vi "G#Object_ExternalCreateProcess.vi"(0 "occurrence":refnum<k4>, 5 "error in (no error)":errorcluster) -> (19 "error out":errorcluster)   [LabVIEW 2020, in "G#Object.lvclass"]
doc: "This is an external create process that will create an own all objects. It is stopped when running the garbage collector."
uses:
  <vilib>/addons/_AddQ/G#Object/G#Object.lvclass
  <vilib>/addons/_AddQ/G#Object/utils/G#Object_Event.ctl
  <vilib>/addons/_AddQ/G#Object/utils/G#Object_EventType.ctl
  <vilib>/addons/_AddQ/G#Object/utils/G#Object_ObjectInfoType.ctl
  <vilib>/addons/_AddQ/G#Object/utils/G#Object_CreateMethod.ctl
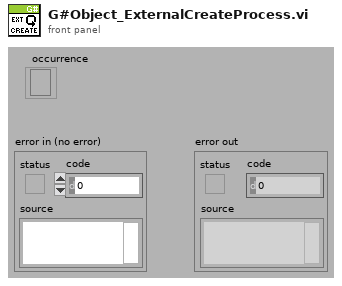
[diagram p1: front panel]
types:
  T1 = typedef "G#Object.lvclass/G#Object_Event.ctl" = cluster{"EventType":T2, "ObjectInfo":T3, "Ref":refnum<class "G#Object.lvclass">, "Time Stamp":timestamp, "LogText":string, "Parameters":variant[]}
  T2 = typedef "G#Object.lvclass/G#Object_EventType.ctl" = enum16{"Created new", "Looked up existing", "Deleted", "Forced delete", "Not deleted", "Garbage collected", "Cleared", "User", "Error", "External create object", "External create class attributes", "Created class attributes", "Run constructor", "Run constructor done", "Run open method", "Run open method done"}
  T3 = typedef "G#Object.lvclass/G#Object_ObjectInfoType.ctl" = cluster{"ObjectName":string, "ObjectID":u32, "Users":i32, "Counter":bool, "AttributeRefs":u32[], "FullClassName":string, "ClassName":string, "CreateMethod":T4, "GenericDestructorExists":bool, "Owner":string}
  T4 = typedef "G#Object.lvclass/G#Object_CreateMethod.ctl" = enum16{"Create", "Create or look up existing", "Look up existing"}
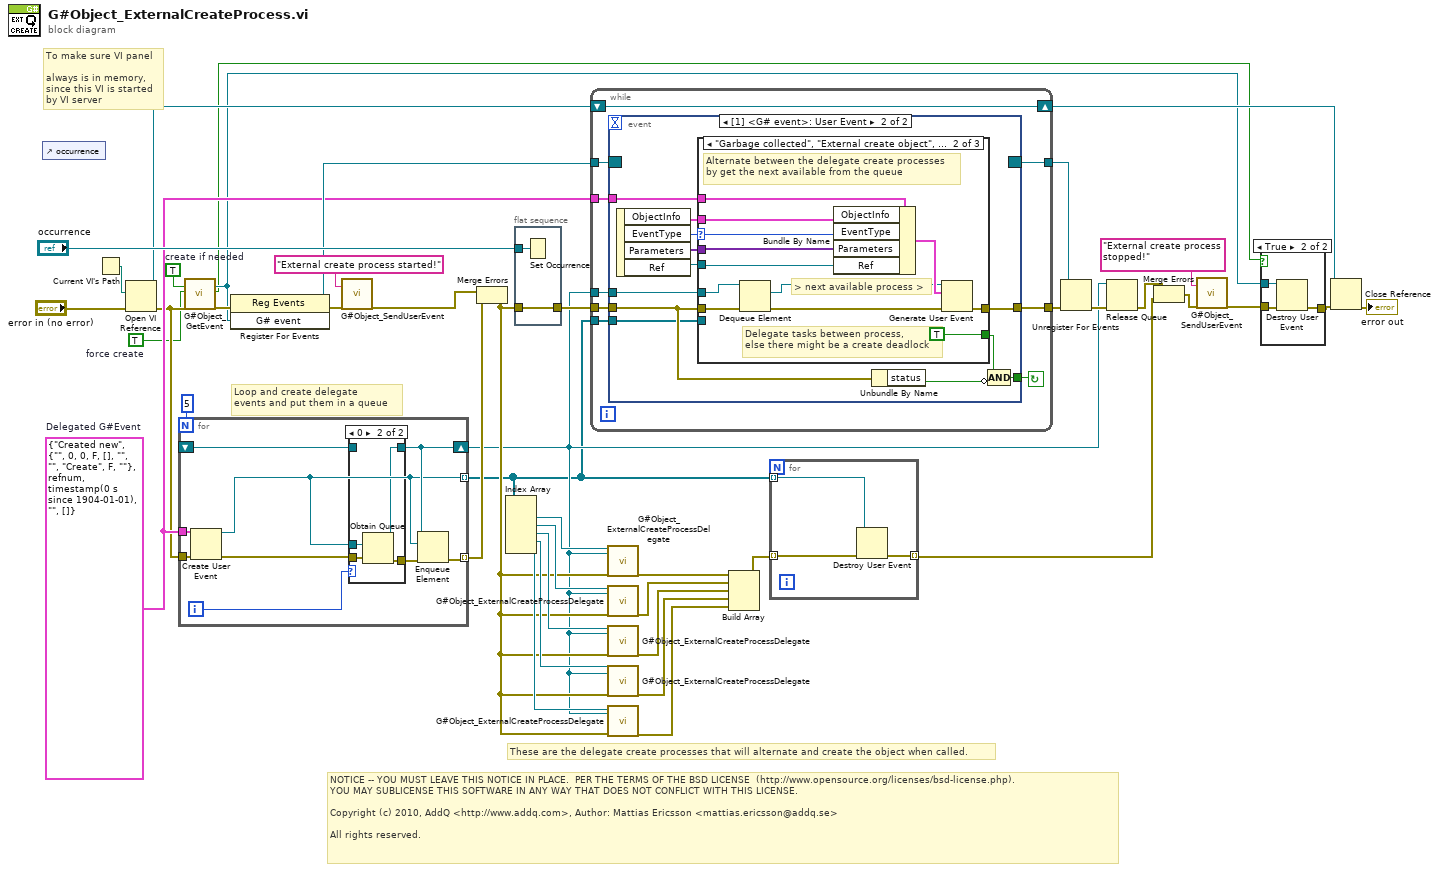
[diagram p0: block diagram]
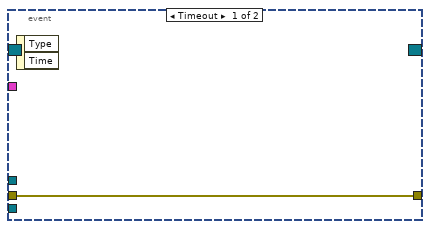
[diagram p4: hidden frame]
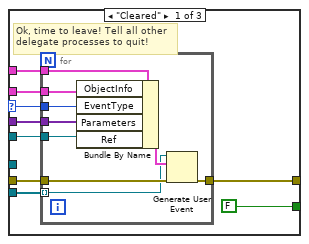
[diagram p5: hidden frame]
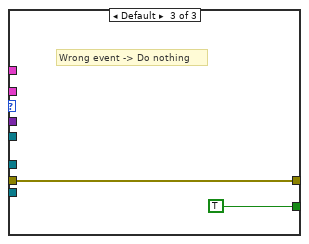
[diagram p6: hidden frame]
diagram:
  w2 = TRUE  # force create
  w30 = T1 {"EventType"=enum."Created new", "ObjectInfo"={"ObjectName"="", "ObjectID"=0, "Users"=0, "Counter"=FALSE, "AttributeRefs"=[], "FullClassName"="", "ClassName"="", "CreateMethod"=enum."Create", "GenericDestructorExists"=FALSE, "Owner"=""}, "Ref"=refnum, "Time Stamp"=timestamp(0 s since 1904-01-01), "LogText"="", "Parameters"=[]}  # Delegated G#Event
  w40 = TRUE  # create if needed
  # "Loop and create delegate\nevents and put them in a queue"
  # "These are the delegate create processes that will alternate and create the object when called."
  # "To make sure VI panel\n\nalways is in memory,\nsince this VI is started\nby VI server"
  # "NOTICE -- YOU MUST LEAVE THIS NOTICE IN PLACE.  PER THE TERMS OF THE BSD LICENSE  (http://www.opensource.org/licenses/bsd-license.php).\nYOU MAY SUBLICENSE THIS SOFTWARE IN ANY WAY THAT DOES NOT CONFLICT WITH THIS LICENSE.\n\nCopyright (c) 2010, AddQ <http://www.addq.com>, Author: Mattias Ericsson <mattias.ericsson@addq.se>\n\nAll rights reserved."
  n1 = control-ref of="occurrence"() -> ()  [unwired: 1 out]
  n2 = Current VI's Path() -> (path=w35:path)
  n3 = Open VI Reference(vi path=w35, error in (no error)="error in (no error)") -> (vi reference=w36:refnum<vi>, error out=w29:errorcluster)  [unwired: 4 in]
  n4 = for {
    N: 5 -> [_]
    tunnel: w30 -> [w52]
    tunnel: w29 -> [w51]
    tunnel: [w46] -> w1 mode=indexing
    tunnel: [w45] -> w24 mode=indexing
    shift-right: [w47] -> w8
    shift-left: _ -> [w49]
    i -> [w50]
    n5 = Create User Event(user event datatype=w52, error in=w51) -> (user event=w46:refnum<user-event>, error out=w44:errorcluster)
    n6 = case shown="0" w50 {
      tunnel: w44 -> [w53 w58]
      tunnel: w46 -> [_ w57]
      tunnel: [w54 w56] -> w47
      tunnel: w49 -> [w54 _]
      tunnel: [w53 w55] -> w48
      frame Default {
      }
      frame 0 {
        n7 = Obtain Queue(element data type=w57, error in (no error)=w58) -> (queue out=w56:refnum<queue>, error out=w55:errorcluster)  [unwired: 3 in, 1 out]
      }
    }
    n8 = Enqueue Element(queue=w47, element=w46, error in (no error)=w48) -> (error out=w45:errorcluster)  [unwired: 1 in, 2 out]
  }
  n9 = call <vilib>:"G#Object_GetEvent.vi"("create if needed (T)"=w40, "force create (F)"=w2, "error in (no error)"=w29) -> ("G# event"=w4:refnum<user-event>, "created new"=w3:bool, "error out"=w39:errorcluster)  [unwired: 12 in, 2 out]
  n10 = register-events(error in=w39, w4) -> (reference out=w37:refnum<event-registration>, error out=w33:errorcluster)  [unwired: 1 in]
  n11 = call <vilib>:"G#Object_SendUserEvent.vi"("text"="External create process started!" ("Text"), "error in (no error)"=w33) -> ("error out"=w28:errorcluster)  [unwired: 16 in, 1 out]
  n12 = Merge Errors(w28, w24) -> (w13:errorcluster)
  n13 = Index Array(array=w1) -> (element #1=w18:refnum<user-event>, element #2=w17:refnum<user-event>, element #3=w16:refnum<user-event>, element #4=w15:refnum<user-event>, element #5=w14:refnum<user-event>)  [unwired: 5 in]
  n14 = flat-sequence {
    tunnel: "occurrence" -> [w60]
    tunnel: w13 -> [w59]
    tunnel: [w59] -> w12
    frame #0 {
      n15 = Set Occurrence(w60) -> ()
    }
  }
  n16 = while {
    tunnel: w12 -> [w69]
    tunnel: [w68] -> w31
    tunnel: w37 -> [w67]
    tunnel: [w66] -> w38
    shift-right: [w65] -> w34
    shift-left: w36 -> [w65]
    tunnel: w30 -> [w63]
    tunnel: w8 -> [w62]
    tunnel: w1 -> [w61]
    stop <- w64 continue-if-true
    n17 = event shown="[1] <G# event>: User Event" {
      selector: w67 -> [_ _]
      dyn-events: [_ _] -> w66
      timeout: _ -> [_ _]
      tunnel: w69 -> [w70 w80]
      tunnel: [w70 w82] -> w68
      tunnel: [_ w77] -> w64
      tunnel: w63 -> [_ w74]
      tunnel: w62 -> [_ w73]
      tunnel: w61 -> [_ w72]
      event Timeout {
        n18 = event-data() -> ()  [unwired: 1 in, 2 out]
      }
      event User Event {
        n19 = event-data() -> ("ObjectInfo"=w75:T3, "EventType"=w81:T2, "Parameters"=w76:variant[], "Ref"=w71:refnum<class "G#Object.lvclass">)  [unwired: 1 in]
        n20 = case shown="\"Garbage collected\", \"External create object\", \"External create class attributes\", \"Run constructor\", \"Run open method\"" w81 {
          selector: w81 -> [w88 w108 _]
          tunnel: w80 -> [w87 w105 w113]
          tunnel: [w90 w111 w113] -> w82
          tunnel: [FALSE TRUE TRUE] -> w78
          tunnel: w76 -> [w84 w107 _]
          tunnel: w75 -> [w85 w109 _]
          tunnel: w74 -> [w89 w110 _]
          tunnel: w73 -> [_ w103 _]
          tunnel: w72 -> [w86 _ _]
          tunnel: w71 -> [w83 w101 _]
          frame "Cleared" {
            # "Ok, time to leave! Tell all other\ndelegate processes to quit!"
            n21 = for {
              tunnel: w87 -> [w100]
              tunnel: [w99] -> w90
              tunnel: w89 -> [w98]
              tunnel: w88 -> [w96]
              tunnel: w86 -> [w95] mode=indexing
              tunnel: w85 -> [w94]
              tunnel: w84 -> [w93]
              tunnel: w83 -> [w92]
              n22 = Bundle By Name(cluster=w98, "ObjectInfo"=w94, "EventType"=w96, "Parameters"=w93, "Ref"=w92) -> (w97:T1)
              n23 = Generate User Event(user event=w95, event data cluster=w97, error in=w100) -> (error out=w99:errorcluster)  [unwired: 1 in, 1 out]
            }
          }
          frame "Garbage collected", "External create object", "External create class attributes", "Run constructor", "Run open method" {
            # "> next available process >"
            # "Delegate tasks between process,\nelse there might be a create deadlock"
            # "Alternate between the delegate create processes\nby get the next available from the queue"
            n24 = Dequeue Element(queue=w103, error in (no error)=w105) -> (element=w102:refnum<user-event>, error out=w104:errorcluster)  [unwired: 1 in, 2 out]
            n25 = Bundle By Name(cluster=w110, "ObjectInfo"=w109, "EventType"=w108, "Parameters"=w107, "Ref"=w101) -> (w106:T1)
            n26 = Generate User Event(user event=w102, event data cluster=w106, error in=w104) -> (error out=w111:errorcluster)  [unwired: 1 in, 1 out]
          }
          frame Default {
            # "Wrong event -> Do nothing"
          }
        }
        n27 = Unbundle By Name(w80) -> ("status"=w79:bool)
        n28 = Compound Arithmetic op=AND(w78, invert w79) -> (w77:bool)
      }
    }
  }
  n29 = call <vilib>:"G#Object_ExternalCreateProcessDelegate.vi"("delegate event out"=w18, "event queue"=w8, "error in (no error)"=w13) -> ("error out"=w25:errorcluster)  [unwired: 16 in]
  n30 = call <vilib>:"G#Object_ExternalCreateProcessDelegate.vi"("delegate event out"=w17, "event queue"=w8, "error in (no error)"=w13) -> ("error out"=w23:errorcluster)  [unwired: 16 in]
  n31 = call <vilib>:"G#Object_ExternalCreateProcessDelegate.vi"("delegate event out"=w16, "event queue"=w8, "error in (no error)"=w13) -> ("error out"=w22:errorcluster)  [unwired: 16 in]
  n32 = call <vilib>:"G#Object_ExternalCreateProcessDelegate.vi"("delegate event out"=w15, "event queue"=w8, "error in (no error)"=w13) -> ("error out"=w21:errorcluster)  [unwired: 16 in]
  n33 = call <vilib>:"G#Object_ExternalCreateProcessDelegate.vi"("delegate event out"=w14, "event queue"=w8, "error in (no error)"=w13) -> ("error out"=w20:errorcluster)  [unwired: 16 in]
  n34 = Build Array(w25, w23, w22, w21, w20) -> (w19:errorcluster[])
  n35 = for {
    tunnel: [w117] -> w26 mode=indexing
    tunnel: w1 -> [w116] mode=indexing
    tunnel: w19 -> [w115] mode=indexing
    n36 = Destroy User Event(user event=w116, error in=w115) -> (error out=w117:errorcluster)
  }
  n37 = Unregister For Events(event registration refnum=w38, error in=w31) -> (error out=w11:errorcluster)
  n38 = Release Queue(queue=w8, error in (no error)=w11) -> (error out=w10:errorcluster)  [unwired: 1 in, 2 out]
  n39 = Merge Errors(w10, w26) -> (w9:errorcluster)
  n40 = call <vilib>:"G#Object_SendUserEvent.vi"("text"="External create process stopped!" ("Text"), "error in (no error)"=w9) -> ("error out"=w6:errorcluster)  [unwired: 16 in, 1 out]
  n41 = case shown="True" w3 {
    tunnel: w6 -> [w118 w121]
    tunnel: [w118 w120] -> w5
    tunnel: w4 -> [_ w119]
    frame False {
    }
    frame True {
      n42 = Destroy User Event(user event=w119, error in=w121) -> (error out=w120:errorcluster)
    }
  }
  n43 = Close Reference(reference=w34, error in (no error)=w5) -> (error out=→"error out":errorcluster)
